vi "A_per_S2T_per_min.vi"(1 "A/sec":dbl format="%.1f") -> (0 "T/min":dbl format="%.4f")   [LabVIEW 2019]
uses:
  PS Comm Globals.vi
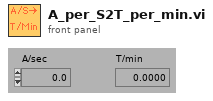
[diagram p1: front panel]
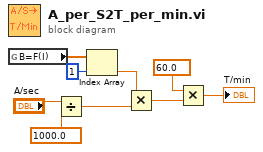
[diagram p0: block diagram]
diagram:
  n1 = global read "PS Comm Globals.vi" "B=F(I)"() -> (w5:dbl[])
  n2 = Divide(x="A/sec", y=1000.0) -> (x/y=w3:dbl)
  n3 = Index Array(array=w5, index=1 ("Index")) -> (element=w2:dbl)
  n4 = Multiply(x=w2, y=w3) -> (x*y=w1:dbl)
  n5 = Multiply(x=60.0, y=w1) -> (x*y=→"T/min":dbl)
